vi "Launch Keypad Dialog Box.vi"(9 "Parameter Name":string, 10 "Reply Transport":refnum<class "ITransport.lvclass">, 11 "Dialog Launcher":refnum<class "IViewable.lvclass">) -> (0 "error out":errorcluster)   [LabVIEW 2015, in "KeypadDialogBox.lvlib" / "KeypadDialogBox.lvclass"]
uses:
  KeypadDialogBox.lvclass
  Framework/IViewable/IViewable/IViewable.lvclass
  Framework/IMediator/ITransport/ITransport.lvclass
  KeypadDialogBox.lvclass/KeypadDialogBox.ctl
  <vilib>/ActorFramework/Actor/Actor.lvclass/Actor.ctl
  <vilib>/ActorFramework/Message Enqueuer/Message Enqueuer.lvclass/Message Enqueuer.ctl
  Framework/IViewable/IViewable Messages/Launch Dialog Box Msg/Launch Dialog Box Msg.lvclass/Launch Dialog Box Msg.ctl
  <vilib>/ActorFramework/Message Enqueuer/Init from Existing Queue.vi
  <vilib>/ActorFramework/Message Enqueuer/Enqueue.vi
  <vilib>/ActorFramework/Message Priority Queue/Priority Enqueue.vi
  <vilib>/ActorFramework/Message Enqueuer/Message Enqueuer.lvclass
  Framework/IViewable/IViewable Messages/Launch Dialog Box Msg/Launch Dialog Box Msg.lvclass
  <vilib>/ActorFramework/Actor/Actor.lvclass
panel:
  in  "error in (no error)":errorcluster
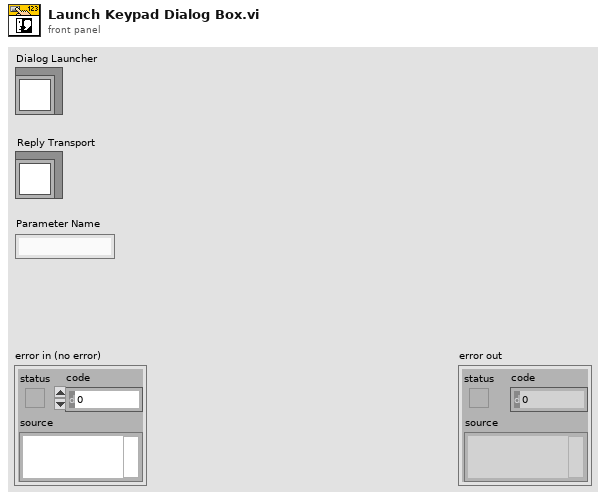
[diagram p1: front panel]
types:
  T1 = enum32{"Invalid", "Default", "Floating", "Floating/Auto-Hide", "Modal"}
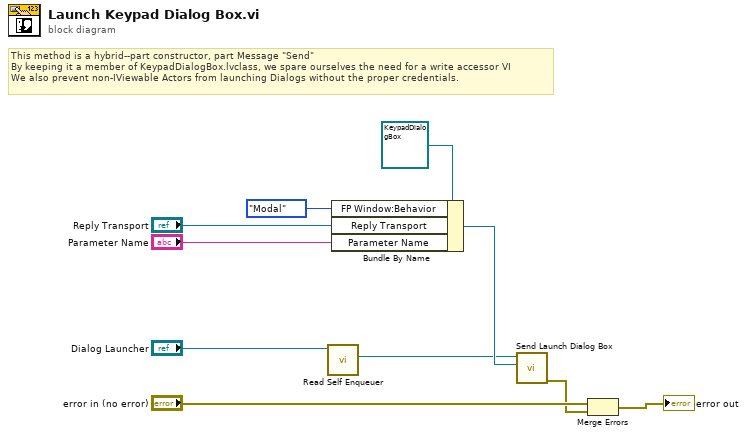
[diagram p0: block diagram]
diagram:
  # "This method is a hybrid--part constructor, part Message \"Send\"\nBy keeping it a member of KeypadDialogBox.lvclass, we spare ourselves the need for a write accessor VI\nWe also prevent non-IViewable Actors from launching Dialogs without the proper credentials."
  n1 = call <vilib>:"Read Self Enqueuer.vi"("Actor"="Dialog Launcher") -> ("Self Enqueuer"=w4:refnum<class "Message Enqueuer.lvclass">)  [unwired: 10 in]
  n2 = Bundle By Name(cluster=refnum<class "KeypadDialogBox.lvclass"> refnum ("OneButtonDialogBox in"), "FP Window:Behavior"=T1."Modal", "Reply Transport"="Reply Transport", "Parameter Name"="Parameter Name") -> (w5:refnum<class "KeypadDialogBox.lvclass">)
  n3 = call "Send Launch Dialog Box.vi"("DialogBox"=w5, "Message Enqueuer"=w4) -> ("error out"=w6:errorcluster)  [unwired: 8 in, 1 out]
  n4 = Merge Errors("error in (no error)", w6) -> (→"error out":errorcluster)
